vi "Create or Replace VI From Template.vi"(8 "error in (no error)":errorcluster, 9 "vi name":string, 10 "template vi path":path, 11 "library in":refnum<vi>) -> (0 "error out":errorcluster, 1 "existing vi":bool, 2 "vi":refnum<vi>, 3 "Library out":refnum<vi>)   [LabVIEW 2019, in "gRPC Template Creation Utility.lvlib"]
uses:
  gRPC Template Creation Utility.lvlib
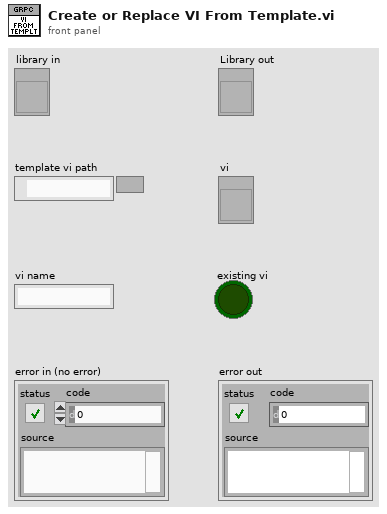
[diagram p1: front panel]
types:
  T1 = enum16{"Invalid Wire Rule", "Required", "Recommended", "Optional", "Dynamic Dispatch"}[]
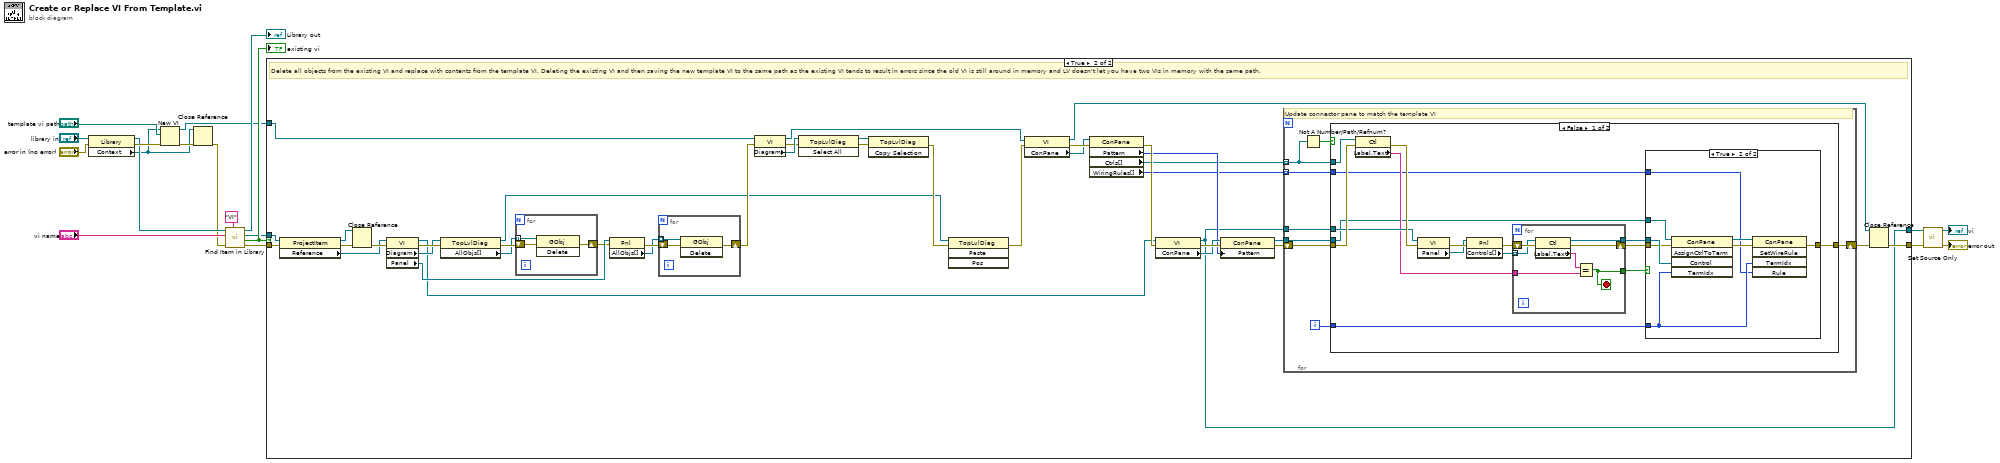
[diagram p0: block diagram]
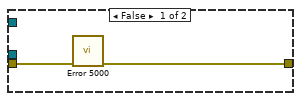
[diagram p3: hidden frame]
diagram:
  n1 = property class="Library"(reference="library in", error in="error in (no error)") -> (reference out=w10:refnum<vi>, error out=w19:errorcluster, "Context"=w1:refnum<vi>)
  n2 = New VI(8:w19, 10:"template vi path", 11:w1) -> (0:w4:errorcluster, 3:w3:refnum<vi>)  [unwired: 4 in]
  n3 = Close Reference(reference=w1, error in (no error)=w4) -> (error out=w2:errorcluster)
  n4 = call "Find Item in Library.vi"("Item Type"="VI", "error in (no error)"=w2, "Item Name"="vi name", "Library item in"=w10) -> ("error out"=w12:errorcluster, "Found?"=w13:bool, "Project Item (Library Item)"=w11:refnum<vi>, "Library item out"=→"Library out":refnum<vi>)  [unwired: 4 in]
  "existing vi" <- w13
  n5 = case shown="True" w13 {
    tunnel: w12 -> [w21 w60]
    tunnel: w11 -> [_ w59]
    tunnel: w3 -> [w20 w58]
    tunnel: [w21 w38] -> w9
    tunnel: [w20 w37] -> w8
    frame False {
      # "No pre-existing VI. Use the new VI that was copied from the template."
    }
    frame True {
      # "Delete all objects from the existing VI and replace with contents from the template VI. Deleting the existing VI and then saving the new template VI to the same path as the existing VI tends to result in errors since the old VI is still around in memory and LV doesn't let you have two VIs in memory with the same path."
      n6 = property class="ProjectItem"(reference=w59, error in=w60) -> (reference out=w35:refnum<vi>, error out=w36:errorcluster, "Reference"=w33:refnum<vi>)
      n7 = Close Reference(reference=w35, error in (no error)=w36) -> (error out=w34:errorcluster)
      n8 = property class="VI"(reference=w33, error in=w34) -> (reference out=w26:refnum<vi>, error out=w32:errorcluster, "Diagram"=w31:refnum<vi>, "Panel"=w30:refnum<vi>)
      n9 = property class="TopLvlDiag"(reference=w31, error in=w32) -> (reference out=w27:refnum<vi>, error out=w23:errorcluster, "AllObjs[]"=w22:refnum<vi>[])
      n10 = for {
        tunnel: w22 -> [w63] mode=indexing
        shift-right: [w61] -> w24
        shift-left: w23 -> [w62]
        n11 = invoke class="GObj" method="Delete"(reference=w63, error in=w62) -> (error out=w61:errorcluster)  [unwired: 1 in, 2 out]
      }
      n12 = property class="Pnl"(reference=w30, error in=w24) -> (error out=w29:errorcluster, "AllObjs[]"=w25:refnum<vi>[])  [unwired: 1 out]
      n13 = for {
        tunnel: w25 -> [w108] mode=indexing
        shift-right: [w106] -> w53
        shift-left: w29 -> [w107]
        n14 = invoke class="GObj" method="Delete"(reference=w108, error in=w107) -> (error out=w106:errorcluster)  [unwired: 1 in, 2 out]
      }
      n15 = property class="VI"(reference=w58, error in=w53) -> (reference out=w52:refnum<vi>, error out=w54:errorcluster, "Diagram"=w57:refnum<vi>)
      n16 = invoke class="TopLvlDiag" method="Select All"(reference=w57, error in=w54) -> (reference out=w56:refnum<vi>, error out=w55:errorcluster)  [unwired: 1 in, 1 out]
      n17 = invoke class="TopLvlDiag" method="Copy Selection"(reference=w56, error in=w55) -> (error out=w28:errorcluster)  [unwired: 1 in, 2 out]
      n18 = invoke class="TopLvlDiag" method="Paste"(reference=w27, error in=w28) -> (error out=w51:errorcluster)  [unwired: 2 in, 3 out]
      n19 = property class="VI"(reference=w52, error in=w51) -> (reference out=w39:refnum<vi>, error out=w50:errorcluster, "ConPane"=w49:refnum<vi>)
      n20 = property class="ConPane"(reference=w49, error in=w50) -> (error out=w47:errorcluster, "Pattern"=w45:u32, "Ctrls[]"=w44:refnum<vi>[], "WiringRules[]"=w43:T1)  [unwired: 1 out]
      n21 = property class="VI"(reference=w26, error in=w47) -> (reference out=w37:refnum<vi>, error out=w48:errorcluster, "ConPane"=w46:refnum<vi>)
      n22 = property class="ConPane"(reference=w46, error in=w48, "Pattern"=w45) -> (reference out=w41:refnum<vi>, error out=w42:errorcluster)
      n23 = for {
        tunnel: w44 -> [w68] mode=indexing
        tunnel: w43 -> [w64] mode=indexing
        tunnel: w41 -> [w66]
        tunnel: w37 -> [w67]
        shift-right: [w69] -> w40
        shift-left: w42 -> [w70]
        i -> [w65]
        # "Update connector pane to match the template VI"
        n24 = Not A Number/Path/Refnum?(number/path/refnum=w68) -> (NaN/Path/Refnum?=w71:bool)
        n25 = case shown="False" w71 {
          tunnel: w70 -> [w86 w105]
          tunnel: [w76 w105] -> w69
          tunnel: w68 -> [w87 _]
          tunnel: w67 -> [w84 _]
          tunnel: w66 -> [w73 _]
          tunnel: w65 -> [w74 _]
          tunnel: w64 -> [w72 _]
          frame False {
            n26 = property class="Ctl"(reference=w87, error in=w86) -> (error out=w85:errorcluster, "Label.Text"=w79:string)  [unwired: 1 out]
            n27 = property class="VI"(reference=w84, error in=w85) -> (error out=w83:errorcluster, "Panel"=w82:refnum<vi>)  [unwired: 1 out]
            n28 = property class="Pnl"(reference=w82, error in=w83) -> (error out=w80:errorcluster, "Controls[]"=w81:refnum<vi>[])  [unwired: 1 out]
            n29 = for {
              tunnel: w81 -> [w103] mode=indexing
              shift-right: [w99] -> w77
              shift-left: w80 -> [w104]
              tunnel: w79 -> [w101]
              tunnel: [w100] -> w75
              tunnel: [w98] -> w78
              stop <- w98 stop-if-true
              n30 = property class="Ctl"(reference=w103, error in=w104) -> (reference out=w100:refnum<vi>, error out=w99:errorcluster, "Label.Text"=w102:string)
              n31 = Equal?(x=w102, y=w101) -> (x = y?=w98:bool)
            }
            n32 = case shown="True" w78 {
              tunnel: w77 -> [w89 w95]
              tunnel: [w88 w91] -> w76
              tunnel: w75 -> [_ w97]
              tunnel: w74 -> [_ w92]
              tunnel: w73 -> [_ w96]
              tunnel: w72 -> [_ w90]
              frame False {
                n33 = call "Error 5000.vi"("error in (no error)"=w89) -> ("error out"=w88:errorcluster)  [unwired: 10 in]
              }
              frame True {
                n34 = invoke class="ConPane" method="AssignCtrlToTerm"(reference=w96, error in=w95, "Control"=w97, "TermIdx"=w92) -> (reference out=w94:refnum<vi>, error out=w93:errorcluster)  [unwired: 1 in, 3 out]
                n35 = invoke class="ConPane" method="SetWireRule"(reference=w94, error in=w93, "TermIdx"=w92, "Rule"=w90) -> (error out=w91:errorcluster)  [unwired: 1 in, 4 out]
              }
            }
          }
          frame True {
          }
        }
      }
      n36 = Close Reference(reference=w39, error in (no error)=w40) -> (error out=w38:errorcluster)
    }
  }
  n37 = call "Set Source Only.vi"("error in (no error)"=w9, "VI in"=w8) -> ("error out"=→"error out":errorcluster, "VI out"=→"vi":refnum<vi>)  [unwired: 8 in]
